vi "rsidr_core_global.vi"() -> ()   [LabVIEW 2020, in "Rohde&Schwarz CMWXP NR FR1 Measurement.lvlib"] (continued)
"Command"="FETC:NRS:MEAS{instance}:MEV:MERR:CURR?", "Access"=enum."Read Only", "Range Table"="", "Read Callback"="", "Write Callback"="", "Range Callback"="", "Check Callback"="", "Rngtable Callback"="", "Coerce Callback"="", "Supported Models"="", "Instrument Options"="", "Check Status Callback"="", "Flags"=0, "Help"="Returns the values of the magnitude error bar graphs for the OFDM symbols in the measured slot. The results of the current bar graph are retrieved.\nThere is one pair of magnitude error values per OFDM symbol, returned in the following order:\n<Reliability>, {<Low>, <High>}symbol 0, {<Low>, <High>}symbol 1, ...\n\nReturn values:\n<Reliability>\n decimal\n\n<Low>\n float\nMagnitude error value for low EVM window position.\nDefault unit:  %\n\n<High>\n float\nMagnitude error value for high EVM window position.\nDefault unit:  %\n\nAvailable Repeated Capabilities:\ninstance: i0, i1, i2, i3, i4, i5, i6, i7, i8, i9, i10, i11, i12, i13, i14, i15, i16, i17, i18, i19, i20, i21, i22, i23, i24, i25, i26, i27, i28, i29, i30, i31, i32\r\n\nRemote-control command(s):\nFETCh:NRSub:MEAS<i>:MEValuation:MERRor:CURRent?"}, {"Level"=4, "Class Only"=FALSE, "Identifier"="RSCMWXPNRFR1M_ATTR_FETCH_MULTI_EVAL_MEAS_MAGNITUDE_ERROR_AVERAGE_RESULTS", "Descriptive Name"="Fetch Multi Eval Meas Magnitude Error Average Results", "Data Type"=enum."RawString", "Command"="FETC:NRS:MEAS{instance}:MEV:MERR:AVER?", "Access"=enum."Read Only", "Range Table"="", "Read Callback"="", "Write Callback"="", "Range Callback"="", "Check Callback"="", "Rngtable Callback"="", "Coerce Callback"="", "Supported Models"="", "Instrument Options"="", "Check Status Callback"="", "Flags"=0, "Help"="Returns the values of the magnitude error bar graphs for the OFDM symbols in the measured slot. The results of the average bar graph are retrieved.\nThere is one pair of magnitude error values per OFDM symbol, returned in the following order:\n<Reliability>, {<Low>, <High>}symbol 0, {<Low>, <High>}symbol 1, ...\n\nReturn values:\n<Reliability>\n decimal\n\n<Low>\n float\nMagnitude error value for low EVM window position.\nDefault unit:  %\n\n<High>\n float\nMagnitude error value for high EVM window position.\nDefault unit:  %\n\nAvailable Repeated Capabilities:\ninstance: i0, i1, i2, i3, i4, i5, i6, i7, i8, i9, i10, i11, i12, i13, i14, i15, i16, i17, i18, i19, i20, i21, i22, i23, i24, i25, i26, i27, i28, i29, i30, i31, i32\r\n\nRemote-control command(s):\nFETCh:NRSub:MEAS<i>:MEValuation:MERRor:AVERage?"}, {"Level"=4, "Class Only"=FALSE, "Identifier"="RSCMWXPNRFR1M_ATTR_FETCH_MULTI_EVAL_MEAS_MAGNITUDE_ERROR_MAXIMUM_RESULTS", "Descriptive Name"="Fetch Multi Eval Meas Magnitude Error Maximum Results", "Data Type"=enum."RawString", "Command"="FETC:NRS:MEAS{instance}:MEV:MERR:MAX?", "Access"=enum."Read Only", "Range Table"="", "Read Callback"="", "Write Callback"="", "Range Callback"="", "Check Callback"="", "Rngtable Callback"="", "Coerce Callback"="", "Supported Models"="", "Instrument Options"="", "Check Status Callback"="", "Flags"=0, "Help"="Returns the values of the magnitude error bar graphs for the OFDM symbols in the measured slot. The results of the maximum bar graph are retrieved.\nThere is one pair of magnitude error values per OFDM symbol, returned in the following order:\n<Reliability>, {<Low>, <High>}symbol 0, {<Low>, <High>}symbol 1, ...\n\nReturn values:\n<Reliability>\n decimal\n\n<Low>\n float\nMagnitude error value for low EVM window position.\nDefault unit:  %\n\n<High>\n float\nMagnitude error value for high EVM window position.\nDefault unit:  %\n\nAvailable Repeated Capabilities:\ninstance: i0, i1, i2, i3, i4, i5, i6, i7, i8, i9, i10, i11, i12, i13, i14, i15, i16, i17, i18, i19, i20, i21, i22, i23, i24, i25, i26, i27, i28, i29, i30, i31, i32\r\n\nRemote-control command(s):\nFETCh:NRSub:MEAS<i>:MEValuation:MERRor:MAXimum?"}, {"Level"=3, "Class Only"=TRUE, "Identifier"="", "Descriptive Name"="Phase Error", "Data Type"=enum."ViInt32", "Command"="", "Access"=enum."Read Only", "Range Table"="", "Read Callback"="", "Write Callback"="", "Range Callback"="", "Check Callback"="", "Rngtable Callback"="", "Coerce Callback"="", "Supported Models"="", "Instrument Options"="", "Check Status Callback"="", "Flags"=0, "Help"="The commands in this class return the contents of the phase error vs OFDM symbol result diagram."}, {"Level"=4, "Class Only"=FALSE, "Identifier"="RSCMWXPNRFR1M_ATTR_READ_MULTI_EVAL_MEAS_PHASE_ERROR_CURRENT_RESULTS", "Descriptive Name"="Read Multi Eval Meas Phase Error Current Results", "Data Type"=enum."RawString", "Command"="READ:NRS:MEAS{instance}:MEV:PERR:CURR?", "Access"=enum."Read Only", "Range Table"="", "Read Callback"="", "Write Callback"="", "Range Callback"="", "Check Callback"="", "Rngtable Callback"="", "Coerce Callback"="", "Supported Models"="", "Instrument Options"="", "Check Status Callback"="", "Flags"=0, "Help"="Returns the values of the phase error bar graphs for the OFDM symbols in the measured slot. The results of the current bar graph are retrieved.\nThere is one pair of phase error values per OFDM symbol, returned in the following order:\n<Reliability>, {<Low>, <High>}symbol 0, {<Low>, <High>}symbol 1, ...\n\nReturn values:\n<Reliability>\n decimal\n\n<Low>\n float\nPhase error value for low EVM window position.\nDefault unit:  deg\n\n<High>\n float\nPhase error value for high EVM window position.\nDefault unit:  deg\n\nAvailable Repeated Capabilities:\ninstance: i0, i1, i2, i3, i4, i5, i6, i7, i8, i9, i10, i11, i12, i13, i14, i15, i16, i17, i18, i19, i20, i21, i22, i23, i24, i25, i26, i27, i28, i29, i30, i31, i32\r\n\nRemote-control command(s):\nREAD:NRSub:MEAS<i>:MEValuation:PERRor:CURRent?"}, {"Level"=4, "Class Only"=FALSE, "Identifier"="RSCMWXPNRFR1M_ATTR_READ_MULTI_EVAL_MEAS_PHASE_ERROR_AVERAGE_RESULTS", "Descriptive Name"="Read Multi Eval Meas Phase Error Average Results", "Data Type"=enum."RawString", "Command"="READ:NRS:MEAS{instance}:MEV:PERR:AVER?", "Access"=enum."Read Only", "Range Table"="", "Read Callback"="", "Write Callback"="", "Range Callback"="", "Check Callback"="", "Rngtable Callback"="", "Coerce Callback"="", "Supported Models"="", "Instrument Options"="", "Check Status Callback"="", "Flags"=0, "Help"="Returns the values of the phase error bar graphs for the OFDM symbols in the measured slot. The results of the average bar graph are retrieved.\nThere is one pair of phase error values per OFDM symbol, returned in the following order:\n<Reliability>, {<Low>, <High>}symbol 0, {<Low>, <High>}symbol 1, ...\n\nReturn values:\n<Reliability>\n decimal\n\n<Low>\n float\nPhase error value for low EVM window position.\nDefault unit:  deg\n\n<High>\n float\nPhase error value for high EVM window position.\nDefault unit:  deg\n\nAvailable Repeated Capabilities:\ninstance: i0, i1, i2, i3, i4, i5, i6, i7, i8, i9, i10, i11, i12, i13, i14, i15, i16, i17, i18, i19, i20, i21, i22, i23, i24, i25, i26, i27, i28, i29, i30, i31, i32\r\n\nRemote-control command(s):\nREAD:NRSub:MEAS<i>:MEValuation:PERRor:AVERage?"}, {"Level"=4, "Class Only"=FALSE, "Identifier"="RSCMWXPNRFR1M_ATTR_READ_MULTI_EVAL_MEAS_PHASE_ERROR_MAXIMUM_RESULTS", "Descriptive Name"="Read Multi Eval Meas Phase Error Maximum Results", "Data Type"=enum."RawString", "Command"="READ:NRS:MEAS{instance}:MEV:PERR:MAX?", "Access"=enum."Read Only", "Range Table"="", "Read Callback"="", "Write Callback"="", "Range Callback"="", "Check Callback"="", "Rngtable Callback"="", "Coerce Callback"="", "Supported Models"="", "Instrument Options"="", "Check Status Callback"="", "Flags"=0, "Help"="Returns the values of the phase error bar graphs for the OFDM symbols in the measured slot. The results of the maximum bar graph are retrieved.\nThere is one pair of phase error values per OFDM symbol, returned in the following order:\n<Reliability>, {<Low>, <High>}symbol 0, {<Low>, <High>}symbol 1, ...\n\nReturn values:\n<Reliability>\n decimal\n\n<Low>\n float\nPhase error value for low EVM window position.\nDefault unit:  deg\n\n<High>\n float\nPhase error value for high EVM window position.\nDefault unit:  deg\n\nAvailable Repeated Capabilities:\ninstance: i0, i1, i2, i3, i4, i5, i6, i7, i8, i9, i10, i11, i12, i13, i14, i15, i16, i17, i18, i19, i20, i21, i22, i23, i24, i25, i26, i27, i28, i29, i30, i31, i32\r\n\nRemote-control command(s):\nREAD:NRSub:MEAS<i>:MEValuation:PERRor:MAXimum?"}, {"Level"=4, "Class Only"=FALSE, "Identifier"="RSCMWXPNRFR1M_ATTR_FETCH_MULTI_EVAL_MEAS_PHASE_ERROR_CURRENT_RESULTS", "Descriptive Name"="Fetch Multi Eval Meas Phase Error Current Results", "Data Type"=enum."RawString", "Command"="FETC:NRS:MEAS{instance}:MEV:PERR:CURR?", "Access"=enum."Read Only", "Range Table"="", "Read Callback"="", "Write Callback"="", "Range Callback"="", "Check Callback"="", "Rngtable Callback"="", "Coerce Callback"="", "Supported Models"="", "Instrument Options"="", "Check Status Callback"="", "Flags"=0, "Help"="Returns the values of the phase error bar graphs for the OFDM symbols in the measured slot. The results of the current bar graph are retrieved.\nThere is one pair of phase error values per OFDM symbol, returned in the following order:\n<Reliability>, {<Low>, <High>}symbol 0, {<Low>, <High>}symbol 1, ...\n\nReturn values:\n<Reliability>\n decimal\n\n<Low>\n float\nPhase error value for low EVM window position.\nDefault unit:  deg\n\n<High>\n float\nPhase error value for high EVM window position.\nDefault unit:  deg\n\nAvailable Repeated Capabilities:\ninstance: i0, i1, i2, i3, i4, i5, i6, i7, i8, i9, i10, i11, i12, i13, i14, i15, i16, i17, i18, i19, i20, i21, i22, i23, i24, i25, i26, i27, i28, i29, i30, i31, i32\r\n\nRemote-control command(s):\nFETCh:NRSub:MEAS<i>:MEValuation:PERRor:CURRent?"}, {"Level"=4, "Class Only"=FALSE, "Identifier"="RSCMWXPNRFR1M_ATTR_FETCH_MULTI_EVAL_MEAS_PHASE_ERROR_AVERAGE_RESULTS", "Descriptive Name"="Fetch Multi Eval Meas Phase Error Average Results", "Data Type"=enum."RawString", "Command"="FETC:NRS:MEAS{instance}:MEV:PERR:AVER?", "Access"=enum."Read Only", "Range Table"="", "Read Callback"="", "Write Callback"="", "Range Callback"="", "Check Callback"="", "Rngtable Callback"="", "Coerce Callback"="", "Supported Models"="", "Instrument Options"="", "Check Status Callback"="", "Flags"=0, "Help"="Returns the values of the phase error bar graphs for the OFDM symbols in the measured slot. The results of the average bar graph are retrieved.\nThere is one pair of phase error values per OFDM symbol, returned in the following order:\n<Reliability>, {<Low>, <High>}symbol 0, {<Low>, <High>}symbol 1, ...\n\nReturn values:\n<Reliability>\n decimal\n\n<Low>\n float\nPhase error value for low EVM window position.\nDefault unit:  deg\n\n<High>\n float\nPhase error value for high EVM window position.\nDefault unit:  deg\n\nAvailable Repeated Capabilities:\ninstance: i0, i1, i2, i3, i4, i5, i6, i7, i8, i9, i10, i11, i12, i13, i14, i15, i16, i17, i18, i19, i20, i21, i22, i23, i24, i25, i26, i27, i28, i29, i30, i31, i32\r\n\nRemote-control command(s):\nFETCh:NRSub:MEAS<i>:MEValuation:PERRor:AVERage?"}, {"Level"=4, "Class Only"=FALSE, "Identifier"="RSCMWXPNRFR1M_ATTR_FETCH_MULTI_EVAL_MEAS_PHASE_ERROR_MAXIMUM_RESULTS", "Descriptive Name"="Fetch Multi Eval Meas Phase Error Maximum Results", "Data Type"=enum."RawString", "Command"="FETC:NRS:MEAS{instance}:MEV:PERR:MAX?", "Access"=enum."Read Only", "Range Table"="", "Read Callback"="", "Write Callback"="", "Range Callback"="", "Check Callback"="", "Rngtable Callback"="", "Coerce Callback"="", "Supported Models"="", "Instrument Options"="", "Check Status Callback"="", "Flags"=0, "Help"="Returns the values of the phase error bar graphs for the OFDM symbols in the measured slot. The results of the maximum bar graph are retrieved.\nThere is one pair of phase error values per OFDM symbol, returned in the following order:\n<Reliability>, {<Low>, <High>}symbol 0, {<Low>, <High>}symbol 1, ...\n\nReturn values:\n<Reliability>\n decimal\n\n<Low>\n float\nPhase error value for low EVM window position.\nDefault unit:  deg\n\n<High>\n float\nPhase error value for high EVM window position.\nDefault unit:  deg\n\nAvailable Repeated Capabilities:\ninstance: i0, i1, i2, i3, i4, i5, i6, i7, i8, i9, i10, i11, i12, i13, i14, i15, i16, i17, i18, i19, i20, i21, i22, i23, i24, i25, i26, i27, i28, i29, i30, i31, i32\r\n\nRemote-control command(s):\nFETCh:NRSub:MEAS<i>:MEValuation:PERRor:MAXimum?"}, {"Level"=3, "Class Only"=TRUE, "Identifier"="", "Descriptive Name"="Inband Emission", "Data Type"=enum."ViInt32", "Command"="", "Access"=enum."Read Only", "Range Table"="", "Read Callback"="", "Write Callback"="", "Range Callback"="", "Check Callback"="", "Rngtable Callback"="", "Coerce Callback"="", "Supported Models"="", "Instrument Options"="", "Check Status Callback"="", "Flags"=0, "Help"="The commands in this class return the inband emission results."}, {"Level"=4, "Class Only"=FALSE, "Identifier"="RSCMWXPNRFR1M_ATTR_READ_MULTI_EVAL_MEAS_TRACE_IEM_CURRENT_RESULTS", "Descriptive Name"="Read Multi Eval Meas Trace IEM Current Results", "Data Type"=enum."RawString", "Command"="READ:NRS:MEAS{instance}:MEV:TRAC:IEM?", "Access"=enum."Read Only", "Range Table"="", "Read Callback"="", "Write Callback"="", "Range Callback"="", "Check Callback"="", "Rngtable Callback"="", "Coerce Callback"="", "Supported Models"="", "Instrument Options"="", "Check Status Callback"="", "Flags"=0, "Help"="Returns the values of the inband emissions trace. The current trace is retrieved.\n\nReturn values:\n<Reliability>\n decimal\n\n<Power>\n float\nComma-separated list of power values, one value per resource block\nDefault unit:  dB\n\nAvailable Repeated Capabilities:\ninstance: i0, i1, i2, i3, i4, i5, i6, i7, i8, i9, i10, i11, i12, i13, i14, i15, i16, i17, i18, i19, i20, i21, i22, i23, i24, i25, i26, i27, i28, i29, i30, i31, i32\r\n\nRemote-control command(s):\nREAD:NRSub:MEAS<i>:MEValuation:TRACe:IEMissions[:CURRent]?"}, {"Level"=4, "Class Only"=FALSE, "Identifier"="RSCMWXPNRFR1M_ATTR_READ_MULTI_EVAL_MEAS_TRACE_IEM_AVERAGE_RESULTS", "Descriptive Name"="Read Multi Eval Meas Trace IEM Average Results", "Data Type"=enum."RawString", "Command"="READ:NRS:MEAS{instance}:MEV:TRAC:IEM:AVER?", "Access"=enum."Read Only", "Range Table"="", "Read Callback"="", "Write Callback"="", "Range Callback"="", "Check Callback"="", "Rngtable Callback"="", "Coerce Callback"="", "Supported Models"="", "Instrument Options"="", "Check Status Callback"="", "Flags"=0, "Help"="Returns the values of the inband emissions trace. The average trace is retrieved.\n\nReturn values:\n<Reliability>\n decimal\n\n<Power>\n float\nComma-separated list of power values, one value per resource block\nDefault unit:  dB\n\nAvailable Repeated Capabilities:\ninstance: i0, i1, i2, i3, i4, i5, i6, i7, i8, i9, i10, i11, i12, i13, i14, i15, i16, i17, i18, i19, i20, i21, i22, i23, i24, i25, i26, i27, i28, i29, i30, i31, i32\r\n\nRemote-control command(s):\nREAD:NRSub:MEAS<i>:MEValuation:TRACe:IEMissions:AVERage?"}, {"Level"=4, "Class Only"=FALSE, "Identifier"="RSCMWXPNRFR1M_ATTR_READ_MULTI_EVAL_MEAS_TRACE_IEM_MAXIMUM_RESULTS", "Descriptive Name"="Read Multi Eval Meas Trace IEM Maximum Results", "Data Type"=enum."RawString", "Command"="READ:NRS:MEAS{instance}:MEV:TRAC:IEM:MAX?", "Access"=enum."Read Only", "Range Table"="", "Read Callback"="", "Write Callback"="", "Range Callback"="", "Check Callback"="", "Rngtable Callback"="", "Coerce Callback"="", "Supported Models"="", "Instrument Options"="", "Check Status Callback"="", "Flags"=0, "Help"="Returns the values of the inband emissions trace. The maximum trace is retrieved.\n\nReturn values:\n<Reliability>\n decimal\n\n<Power>\n float\nComma-separated list of power values, one value per resource block\nDefault unit:  dB\n\nAvailable Repeated Capabilities:\ninstance: i0, i1, i2, i3, i4, i5, i6, i7, i8, i9, i10, i11, i12, i13, i14, i15, i16, i17, i18, i19, i20, i21, i22, i23, i24, i25, i26, i27, i28, i29, i30, i31, i32\r\n\nRemote-control command(s):\nREAD:NRSub:MEAS<i>:MEValuation:TRACe:IEMissions:MAXimum?"}, {"Level"=4, "Class Only"=FALSE, "Identifier"="RSCMWXPNRFR1M_ATTR_FETCH_MULTI_EVAL_MEAS_TRACE_IEM_CURRENT_RESULTS", "Descriptive Name"="Fetch Multi Eval Meas Trace IEM Current Results", "Data Type"=enum."RawString", "Command"="FETC:NRS:MEAS{instance}:MEV:TRAC:IEM?", "Access"=enum."Read Only", "Range Table"="", "Read Callback"="", "Write Callback"="", "Range Callback"="", "Check Callback"="", "Rngtable Callback"="", "Coerce Callback"="", "Supported Models"="", "Instrument Options"="", "Check Status Callback"="", "Flags"=0, "Help"="Returns the values of the inband emissions trace. The current trace is retrieved.\n\nReturn values:\n<Reliability>\n decimal\n\n<Power>\n float\nComma-separated list of power values, one value per resource block\nDefault unit:  dB\n\nAvailable Repeated Capabilities:\ninstance: i0, i1, i2, i3, i4, i5, i6, i7, i8, i9, i10, i11, i12, i13, i14, i15, i16, i17, i18, i19, i20, i21, i22, i23, i24, i25, i26, i27, i28, i29, i30, i31, i32\r\n\nRemote-control command(s):\nFETCh:NRSub:MEAS<i>:MEValuation:TRACe:IEMissions[:CURRent]?"}, {"Level"=4, "Class Only"=FALSE, "Identifier"="RSCMWXPNRFR1M_ATTR_FETCH_MULTI_EVAL_MEAS_TRACE_IEM_AVERAGE_RESULTS", "Descriptive Name"="Fetch Multi Eval Meas Trace IEM Average Results", "Data Type"=enum."RawString", "Command"="FETC:NRS:MEAS{instance}:MEV:TRAC:IEM:AVER?", "Access"=enum."Read Only", "Range Table"="", "Read Callback"="", "Write Callback"="", "Range Callback"="", "Check Callback"="", "Rngtable Callback"="", "Coerce Callback"="", "Supported Models"="", "Instrument Options"="", "Check Status Callback"="", "Flags"=0, "Help"="Returns the values of the inband emissions trace. The average trace is retrieved.\n\nReturn values:\n<Reliability>\n decimal\n\n<Power>\n float\nComma-separated list of power values, one value per resource block\nDefault unit:  dB\n\nAvailable Repeated Capabilities:\ninstance: i0, i1, i2, i3, i4, i5, i6, i7, i8, i9, i10, i11, i12, i13, i14, i15, i16, i17, i18, i19, i20, i21, i22, i23, i24, i25, i26, i27, i28, i29, i30, i31, i32\r\n\nRemote-control command(s):\nFETCh:NRSub:MEAS<i>:MEValuation:TRACe:IEMissions:AVERage?"}, {"Level"=4, "Class Only"=FALSE, "Identifier"="RSCMWXPNRFR1M_ATTR_FETCH_MULTI_EVAL_MEAS_TRACE_IEM_MAXIMUM_RESULTS", "Descriptive Name"="Fetch Multi Eval Meas Trace IEM Maximum Results", "Data Type"=enum."RawString", "Command"="FETC:NRS:MEAS{instance}:MEV:TRAC:IEM:MAX?", "Access"=enum."Read Only", "Range Table"="", "Read Callback"="", "Write Callback"="", "Range Callback"="", "Check Callback"="", "Rngtable Callback"="", "Coerce Callback"="", "Supported Models"="", "Instrument Options"="", "Check Status Callback"="", "Flags"=0, "Help"="Returns the values of the inband emissions trace. The maximum trace is retrieved.\n\nReturn values:\n<Reliability>\n decimal\n\n<Power>\n float\nComma-separated list of power values, one value per resource block\nDefault unit:  dB\n\nAvailable Repeated Capabilities:\ninstance: i0, i1, i2, i3, i4, i5, i6, i7, i8, i9, i10, i11, i12, i13, i14, i15, i16, i17, i18, i19, i20, i21, i22, i23, i24, i25, i26, i27, i28, i29, i30, i31, i32\r\n\nRemote-control command(s):\nFETCh:NRSub:MEAS<i>:MEValuation:TRACe:IEMissions:MAXimum?"}, {"Level"=4, "Class Only"=FALSE, "Identifier"="RSCMWXPNRFR1M_ATTR_READ_MULTI_EVAL_MEAS_TRACE_IEM_LIMIT", "Descriptive Name"="Read Multi Eval Meas Trace IEM Limit", "Data Type"=enum."RawString", "Command"="READ:NRS:MEAS{instance}:MEV:TRAC:IEM:LIM?", "Access"=enum."Read Only", "Range Table"="", "Read Callback"="", "Write Callback"="", "Range Callback"="", "Check Callback"="", "Rngtable Callback"="", "Coerce Callback"="", "Supported Models"="", "Instrument Options"="", "Check Status Callback"="", "Flags"=0, "Help"="Returns the values of the inband emissions limit line.\n\nReturn values:\n<Reliability>\n decimal\n\n<Limit>\n float\nComma-separated list of limit values, one value per resource block\nDefault unit:  dB\n\nAvailable Repeated Capabilities:\ninstance: i0, i1, i2, i3, i4, i5, i6, i7, i8, i9, i10, i11, i12, i13, i14, i15, i16, i17, i18, i19, i20, i21, i22, i23, i24, i25, i26, i27, i28, i29, i30, i31, i32\r\n\nRemote-control command(s):\nREAD:NRSub:MEAS<i>:MEValuation:TRACe:IEMissions:LIMit?"}, {"Level"=4, "Class Only"=FALSE, "Identifier"="RSCMWXPNRFR1M_ATTR_FETCH_MULTI_EVAL_MEAS_TRACE_IEM_LIMIT", "Descriptive Name"="Fetch Multi Eval Meas Trace IEM Limit", "Data Type"=enum."RawString", "Command"="FETC:NRS:MEAS{instance}:MEV:TRAC:IEM:LIM?", "Access"=enum."Read Only", "Range Table"="", "Read Callback"="", "Write Callback"="", "Range Callback"="", "Check Callback"="", "Rngtable Callback"="", "Coerce Callback"="", "Supported Models"="", "Instrument Options"="", "Check Status Callback"="", "Flags"=0, "Help"="Returns the values of the inband emissions limit line.\n\nReturn values:\n<Reliability>\n decimal\n\n<Limit>\n float\nComma-separated list of limit values, one value per resource block\nDefault unit:  dB\n\nAvailable Repeated Capabilities:\ninstance: i0, i1, i2, i3, i4, i5, i6, i7, i8, i9, i10, i11, i12, i13, i14, i15, i16, i17, i18, i19, i20, i21, i22, i23, i24, i25, i26, i27, i28, i29, i30, i31, i32\r\n\nRemote-control command(s):\nFETCh:NRSub:MEAS<i>:MEValuation:TRACe:IEMissions:LIMit?"}, {"Level"=4, "Class Only"=FALSE, "Identifier"="RSCMWXPNRFR1M_ATTR_FETCH_MULTI_EVAL_MEAS_IEM_MARGIN_CURRENT_RESULTS", "Descriptive Name"="Fetch Multi Eval Meas IEM Margin Current Results", "Data Type"=enum."RawString", "Command"="FETC:NRS:MEAS{instance}:MEV:IEM:MARG:CURR?", "Access"=enum."Read Only", "Range Table"="", "Read Callback"="", "Write Callback"="", "Range Callback"="", "Check Callback"="", "Rngtable Callback"="", "Coerce Callback"="", "Supported Models"="", "Instrument Options"="", "Check Status Callback"="", "Flags"=0, "Help"="Return the current limit line margin results. The current margin indicates the minimum (vertical) distance between the inband emissions limit line and the current trace. A negative result indicates that the limit is exceeded. The average, extreme and standard deviation values are calculated from the current margins. The margin results cannot be displayed at the GUI.\n\nReturn values:\n<Reliability>\n decimal\n\n<OutOfTolerance>\n decimal\nOut of tolerance result, i.e. percentage of measurement intervals of the statistic count for modulation measurements exceeding the specified modulation limits.\nDefault unit:  %\n\n<Margin>\n float\nMargin over all non-allocated RBs (scope of general limit component)\nDefault unit:  dB\n\n<IQImage>\n float\nMargin at image frequencies of allocated RBs (scope of IQ image limit component)\nDefault unit:  dB\n\n<CarrLeakage>\n float\nMargin at the carrier frequency (scope of IQ offset limit component)\nDefault unit:  dB\n\nAvailable Repeated Capabilities:\ninstance: i0, i1, i2, i3, i4, i5, i6, i7, i8, i9, i10, i11, i12, i13, i14, i15, i16, i17, i18, i19, i20, i21, i22, i23, i24, i25, i26, i27, i28, i29, i30, i31, i32\r\n\nRemote-control command(s):\nFETCh:NRSub:MEAS<i>:MEValuation:IEMission:MARGin:CURRent?"}, {"Level"=4, "Class Only"=FALSE, "Identifier"="RSCMWXPNRFR1M_ATTR_FETCH_MULTI_EVAL_MEAS_IEM_MARGIN_AVERAGE_RESULTS", "Descriptive Name"="Fetch Multi Eval Meas IEM Margin Average Results", "Data Type"=enum."RawString", "Command"="FETC:NRS:MEAS{instance}:MEV:IEM:MARG:AVER?", "Access"=enum."Read Only", "Range Table"="", "Read Callback"="", "Write Callback"="", "Range Callback"="", "Check Callback"="", "Rngtable Callback"="", "Coerce Callback"="", "Supported Models"="", "Instrument Options"="", "Check Status Callback"="", "Flags"=0, "Help"="Return the average limit line margin results. The current margin indicates the minimum (vertical) distance between the inband emissions limit line and the current trace. A negative result indicates that the limit is exceeded. The average, extreme and standard deviation values are calculated from the current margins. The margin results cannot be displayed at the GUI.\n\nReturn values:\n<Reliability>\n decimal\n\n<OutOfTolerance>\n decimal\nOut of tolerance result, i.e. percentage of measurement intervals of the statistic count for modulation measurements exceeding the specified modulation limits.\nDefault unit:  %\n\n<Margin>\n float\nMargin over all non-allocated RBs (scope of general limit component)\nDefault unit:  dB\n\n<IQImage>\n float\nMargin at image frequencies of allocated RBs (scope of IQ image limit component)\nDefault unit:  dB\n\n<CarrLeakage>\n float\nMargin at the carrier frequency (scope of IQ offset limit component)\nDefault unit:  dB\n\nAvailable Repeated Capabilities:\ninstance: i0, i1, i2, i3, i4, i5, i6, i7, i8, i9, i10, i11, i12, i13, i14, i15, i16, i17, i18, i19, i20, i21, i22, i23, i24, i25, i26, i27, i28, i29, i30, i31, i32\r\n\nRemote-control command(s):\nFETCh:NRSub:MEAS<i>:MEValuation:IEMission:MARGin:AVERage?"}, {"Level"=4, "Class Only"=FALSE, "Identifier"="RSCMWXPNRFR1M_ATTR_FETCH_MULTI_EVAL_MEAS_IEM_MARGIN_EXTREME_RESULTS", "Descriptive Name"="Fetch Multi Eval Meas IEM Margin Extreme Results", "Data Type"=enum."RawString", "Command"="FETC:NRS:MEAS{instance}:MEV:IEM:MARG:EXTR?", "Access"=enum."Read Only", "Range Table"="", "Read Callback"="", "Write Callback"="", "Range Callback"="", "Check Callback"="", "Rngtable Callback"="", "Coerce Callback"="", "Supported Models"="", "Instrument Options"="", "Check Status Callback"="", "Flags"=0, "Help"="Return the extreme limit line margin results. The current margin indicates the minimum (vertical) distance between the inband emissions limit line and the current trace. A negative result indicates that the limit is exceeded. The average, extreme and standard deviation values are calculated from the current margins. The margin results cannot be displayed at the GUI.\n\nReturn values:\n<Reliability>\n decimal\n\n<OutOfTolerance>\n decimal\nOut of tolerance result, i.e. percentage of measurement intervals of the statistic count for modulation measurements exceeding the specified modulation limits.\nDefault unit:  %\n\n<Margin>\n float\nMargin over all non-allocated RBs (scope of general limit component)\nDefault unit:  dB\n\n<IQImage>\n float\nMargin at image frequencies of allocated RBs (scope of IQ image limit component)\nDefault unit:  dB\n\n<CarrLeakage>\n float\nMargin at the carrier frequency (scope of IQ offset limit component)\nDefault unit:  dB\n\nAvailable Repeated Capabilities:\ninstance: i0, i1, i2, i3, i4, i5, i6, i7, i8, i9, i10, i11, i12, i13, i14, i15, i16, i17, i18, i19, i20, i21, i22, i23, i24, i25, i26, i27, i28, i29, i30, i31, i32\r\n\nRemote-control command(s):\nFETCh:NRSub:MEAS<i>:MEValuation:IEMission:MARGin:EXTReme?"}, {"Level"=4, "Class Only"=FALSE, "Identifier"="RSCMWXPNRFR1M_ATTR_FETCH_MULTI_EVAL_MEAS_IEM_MARGIN_STANDARD_DEVIATION_RESULTS", "Descriptive Name"="Fetch Multi Eval Meas IEM Margin Standard Deviation Results", "Data Type"=enum."RawString", "Command"="FETC:NRS:MEAS{instance}:MEV:IEM:MARG:SDEV?", "Access"=enum."Read Only", "Range Table"="", "Read Callback"="", "Write Callback"="", "Range Callback"="", "Check Callback"="", "Rngtable Callback"="", "Coerce Callback"="", "Supported Models"="", "Instrument Options"="", "Check Status Callback"="", "Flags"=0, "Help"="Return the standard deviation limit line margin results. The current margin indicates the minimum (vertical) distance between the inband emissions limit line and the current trace. A negative result indicates that the limit is exceeded.\nThe average, extreme and standard deviation values are calculated from the current margins. The margin results cannot be displayed at the GUI.\n\nReturn values:\n<Reliability>\n decimal\n\n<OutOfTolerance>\n decimal\nOut of tolerance result, i.e. percentage of measurement intervals of the statistic count for modulation measurements exceeding the specified modulation limits.\nDefault unit:  %\n\n<Margin>\n float\nMargin over all non-allocated RBs (scope of general limit component)\nDefault unit:  dB\n\n<IQImage>\n float\nMargin at image frequencies of allocated RBs (scope of IQ image limit component)\nDefault unit:  dB\n\n<CarrLeakage>\n float\nMargin at the carrier frequency (scope of IQ offset limit component)\nDefault unit:  dB\n\nAvailable Repeated Capabilities:\ninstance: i0, i1, i2, i3, i4, i5, i6, i7, i8, i9, i10, i11, i12, i13, i14, i15, i16, i17, i18, i19, i20, i21, i22, i23, i24, i25, i26, i27, i28, i29, i30, i31, i32\r\n\nRemote-control command(s):\nFETCh:NRSub:MEAS<i>:MEValuation:IEMission:MARGin:SDEViation?"}, {"Level"=4, "Class Only"=FALSE, "Identifier"="RSCMWXPNRFR1M_ATTR_FETCH_MULTI_EVAL_MEAS_IEM_MARGIN_RB_INDEX_CURRENT_RESULTS", "Descriptive Name"="Fetch Multi Eval Meas IEM Margin RB Index Current Results", "Data Type"=enum."RawString", "Command"="FETC:NRS:MEAS{instance}:MEV:IEM:MARG:CURR:RBIN?", "Access"=enum."Read Only", "Range Table"="", "Read Callback"="", "Write Callback"="", "Range Callback"="", "Check Callback"="", "Rngtable Callback"="", "Coerce Callback"="", "Supported Models"="", "Instrument Options"="", "Check Status Callback"="", "Flags"=0, "Help"="Return resource block indices for current inband emission margins. At these RB indices, the current, average and extreme margins have been detected.\n\nReturn values:\n<Reliability>\n decimal\n\n<OutOfTolerance>\n decimal\nOut of tolerance result, i.e. percentage of measurement intervals of the statistic count for modulation measurements exceeding the specified modulation limits.\nDefault unit:  %\n\n<RBindex>\n decimal\nResource block index for the general margin (at non-allocated RBs)\n\n<IQImage>\n decimal\nResource block index for the IQ image margin (at image frequencies of allocated RBs)\n\n<CarrLeakage>\n decimal\nResource block index for the carrier leakage margin (at carrier frequency)\n\nAvailable Repeated Capabilities:\ninstance: i0, i1, i2, i3, i4, i5, i6, i7, i8, i9, i10, i11, i12, i13, i14, i15, i16, i17, i18, i19, i20, i21, i22, i23, i24, i25, i26, i27, i28, i29, i30, i31, i32\r\n\nRemote-control command(s):\nFETCh:NRSub:MEAS<i>:MEValuation:IEMission:MARGin:CURRent:RBINdex?"}, {"Level"=4, "Class Only"=FALSE, "Identifier"="RSCMWXPNRFR1M_ATTR_FETCH_MULTI_EVAL_MEAS_IEM_MARGIN_RB_INDEX_AVERAGE_RESULTS", "Descriptive Name"="Fetch Multi Eval Meas IEM Margin RB Index Average Results", "Data Type"=enum."RawString", "Command"="FETC:NRS:MEAS{instance}:MEV:IEM:MARG:AVER:RBIN?", "Access"=enum."Read Only", "Range Table"="", "Read Callback"="", "Write Callback"="", "Range Callback"="", "Check Callback"="", "Rngtable Callback"="", "Coerce Callback"="", "Supported Models"="", "Instrument Options"="", "Check Status Callback"="", "Flags"=0, "Help"="Return resource block indices for average inband emission margins. At these RB indices, the current, average and extreme margins have been detected.\n\nReturn values:\n<Reliability>\n decimal\n\n<OutOfTolerance>\n decimal\nOut of tolerance result, i.e. percentage of measurement intervals of the statistic count for modulation measurements exceeding the specified modulation limits.\nDefault unit:  %\n\n<RBindex>\n decimal\nResource block index for the general margin (at non-allocated RBs)\n\n<IQImage>\n decimal\nResource block index for the IQ image margin (at image frequencies of allocated RBs)\n\n<CarrLeakage>\n decimal\nResource block index for the carrier leakage margin (at carrier frequency)\n\nAvailable Repeated Capabilities:\ninstance: i0, i1, i2, i3, i4, i5, i6, i7, i8, i9, i10, i11, i12, i13, i14, i15, i16, i17, i18, i19, i20, i21, i22, i23, i24, i25, i26, i27, i28, i29, i30, i31, i32\r\n\nRemote-control command(s):\nFETCh:NRSub:MEAS<i>:MEValuation:IEMission:MARGin:AVERage:RBINdex?"}, {"Level"=4, "Class Only"=FALSE, "Identifier"="RSCMWXPNRFR1M_ATTR_FETCH_MULTI_EVAL_MEAS_IEM_MARGIN_RB_INDEX_EXTREME_RESULTS", "Descriptive Name"="Fetch Multi Eval Meas IEM Margin RB Index Extreme Results", "Data Type"=enum."RawString", "Command"="FETC:NRS:MEAS{instance}:MEV:IEM:MARG:EXTR:RBIN?", "Access"=enum."Read Only", "Range Table"="", "Read Callback"="", "Write Callback"="", "Range Callback"="", "Check Callback"="", "Rngtable Callback"="", "Coerce Callback"="", "Supported Models"="", "Instrument Options"="", "Check Status Callback"="", "Flags"=0, "Help"="Return resource block indices for extreme inband emission margins. At these RB indices, the current, average and extreme margins have been detected.\n\nReturn values:\n<Reliability>\n decimal\n\n<OutOfTolerance>\n decimal\nOut of tolerance result, i.e. percentage of measurement intervals of the statistic count for modulation measurements exceeding the specified modulation limits.\nDefault unit:  %\n\n<RBindex>\n decimal\nResource block index for the general margin (at non-allocated RBs)\n\n<IQImage>\n decimal\nResource block index for the IQ image margin (at image frequencies of allocated RBs)\n\n<CarrLeakage>\n decimal\nResource block index for the carrier leakage margin (at carrier frequency)\n\nAvailable Repeated Capabilities:\ninstance: i0, i1, i2, i3, i4, i5, i6, i7, i8, i9, i10, i11, i12, i13, i14, i15, i16, i17, i18, i19, i20, i21, i22, i23, i24, i25, i26, i27, i28, i29, i30, i31, i32\r\n\nRemote-control command(s):\nFETCh:NRSub:MEAS<i>:MEValuation:IEMission:MARGin:EXTReme:RBINdex?"}, {"Level"=3, "Class Only"=TRUE, "Identifier"="", "Descriptive Name"="Equalizer Spectrum Flatness", "Data Type"=enum."ViInt32", "Command"="", "Access"=enum."Read Only", "Range Table"="", "Read Callback"="", "Write Callback"="", "Range Callback"="", "Check Callback"="", "Rngtable Callback"="", "Coerce Callback"="", "Supported Models"="", "Instrument Options"="", "Check Status Callback"="", "Flags"=0, "Help"="The commands in this class return the equalizer spectrum flatness results."}, {"Level"=4, "Class Only"=FALSE, "Identifier"="RSCMWXPNRFR1M_ATTR_READ_MULTI_EVAL_MEAS_TRACE_ES_FLATNESS_RESULTS", "Descriptive Name"="Read Multi Eval Meas Trace ES Flatness Results", "Data Type"=enum."RawString", "Command"="READ:NRS:MEAS{instance}:MEV:TRAC:ESFL?", "Access"=enum."Read Only", "Range Table"="", "Read Callback"="", "Write Callback"="", "Range Callback"="", "Check Callback"="", "Rngtable Callback"="", "Coerce Callback"="", "Supported Models"="", "Instrument Options"="", "Check Status Callback"="", "Flags"=0, "Help"="Returns the values of the equalizer spectrum flatness trace.\n\nReturn values:\n<Reliability>\n decimal\n\n<Power>\n float\nComma-separated list of power values, one value per subcarrier\nFor not allocated subcarriers, NCAP is returned.\nDefault unit:  dB\n\nAvailable Repeated Capabilities:\ninstance: i0, i1, i2, i3, i4, i5, i6, i7, i8, i9, i10, i11, i12, i13, i14, i15, i16, i17, i18, i19, i20, i21, i22, i23, i24, i25, i26, i27, i28, i29, i30, i31, i32\r\n\nRemote-control command(s):\nREAD:NRSub:MEAS<i>:MEValuation:TRACe:ESFLatness?"}, {"Level"=4, "Class Only"=FALSE, "Identifier"="RSCMWXPNRFR1M_ATTR_FETCH_MULTI_EVAL_MEAS_TRACE_ES_FLATNESS_RESULTS", "Descriptive Name"="Fetch Multi Eval Meas Trace ES Flatness Results", "Data Type"=enum."RawString", "Command"="FETC:NRS:MEAS{instance}:MEV:TRAC:ESFL?", "Access"=enum."Read Only", "Range Table"="", "Read Callback"="", "Write Callback"="", "Range Callback"="", "Check Callback"="", "Rngtable Callback"="", "Coerce Callback"="", "Supported Models"="", "Instrument Options"="", "Check Status Callback"="", "Flags"=0, "Help"="Returns the values of the equalizer spectrum flatness trace.\n\nReturn values:\n<Reliability>\n decimal\n\n<Power>\n float\nComma-separated list of power values, one value per subcarrier\nFor not allocated subcarriers, NCAP is returned.\nDefault unit:  dB\n\nAvailable Repeated Capabilities:\ninstance: i0, i1, i2, i3, i4, i5, i6, i7, i8, i9, i10, i11, i12, i13, i14, i15, i16, i17, i18, i19, i20, i21, i22, i23, i24, i25, i26, i27, i28, i29, i30, i31, i32\r\n\nRemote-control command(s):\nFETCh:NRSub:MEAS<i>:MEValuation:TRACe:ESFLatness?"}, {"Level"=4, "Class Only"=FALSE, "Identifier"="RSCMWXPNRFR1M_ATTR_READ_MULTI_EVAL_MEAS_ES_FLATNESS_CURRENT_RESULTS", "Descriptive Name"="Read Multi Eval Meas ES Flatness Current Results", "Data Type"=enum."RawString", "Command"="READ:NRS:MEAS{instance}:MEV:ESFL:CURR?", "Access"=enum."Read Only", "Range Table"="", "Read Callback"="", "Write Callback"="", "Range Callback"="", "Check Callback"="", "Rngtable Callback"="", "Coerce Callback"="", "Supported Models"="", "Instrument Options"="", "Check Status Callback"="", "Flags"=0, "Help"="Return current single value results of the equalizer spectrum flatness measurement.\n\n<1_Reliability>\n decimal\n\n<2_OutOfTol>\n decimal\nOut of tolerance result, i.e. percentage of measurement intervals of the statistic count for modulation measurements exceeding the specified modulation limits.\nDefault unit:  %\n\n<3_Ripple1>\n float\nMax (range 1) - min (range 1)\nDefault unit:  dB\n\n<4_Ripple2>\n float\nMax (range 2) - min (range 2)\nDefault unit:  dB\n\n<5_MaxR1MinR2>\n float\nMax (range 1) - min (range 2)\nDefault unit:  dB\n\n<6_MaxR2MinR1>\n float\nMax (range 2) - min (range 1)\nDefault unit:  dB\n\n<7_MinR1>\n float\nMin (range 1)\nDefault unit:  dB\n\n<8_MaxR1>\n float\nMax (range 1)\nDefault unit:  dB\n\n<9_MinR2>\n float\nMin (range 2)\nDefault unit:  dB\n\n<10_MaxR2>\n float\nMax (range 2)\nDefault unit:  dB\n\nAvailable Repeated Capabilities:\ninstance: i0, i1, i2, i3, i4, i5, i6, i7, i8, i9, i10, i11, i12, i13, i14, i15, i16, i17, i18, i19, i20, i21, i22, i23, i24, i25, i26, i27, i28, i29, i30, i31, i32\r\n\nRemote-control command(s):\nREAD:NRSub:MEAS<i>:MEValuation:ESFLatness:CURRent?"}, {"Level"=4, "Class Only"=FALSE, "Identifier"="RSCMWXPNRFR1M_ATTR_READ_MULTI_EVAL_MEAS_ES_FLATNESS_AVERAGE_RESULTS", "Descriptive Name"="Read Multi Eval Meas ES Flatness Average Results", "Data Type"=enum."RawString", "Command"="READ:NRS:MEAS{instance}:MEV:ESFL:AVER?", "Access"=enum."Read Only", "Range Table"="", "Read Callback"="", "Write Callback"="", "Range Callback"="", "Check Callback"="", "Rngtable Callback"="", "Coerce Callback"="", "Supported Models"="", "Instrument Options"="", "Check Status Callback"="", "Flags"=0, "Help"="Return average single value results of the equalizer spectrum flatness measurement.\n\n<1_Reliability>\n decimal\n\n<2_OutOfTol>\n decimal\nOut of tolerance result, i.e. percentage of measurement intervals of the statistic count for modulation measurements exceeding the specified modulation limits.\nDefault unit:  %\n\n<3_Ripple1>\n float\nMax (range 1) - min (range 1)\nDefault unit:  dB\n\n<4_Ripple2>\n float\nMax (range 2) - min (range 2)\nDefault unit:  dB\n\n<5_MaxR1MinR2>\n float\nMax (range 1) - min (range 2)\nDefault unit:  dB\n\n<6_MaxR2MinR1>\n float\nMax (range 2) - min (range 1)\nDefault unit:  dB\n\n<7_MinR1>\n float\nMin (range 1)\nDefault unit:  dB\n\n<8_MaxR1>\n float\nMax (range 1)\nDefault unit:  dB\n\n<9_MinR2>\n float\nMin (range 2)\nDefault unit:  dB\n\n<10_MaxR2>\n float\nMax (range 2)\nDefault unit:  dB\n\nAvailable Repeated Capabilities:\ninstance: i0, i1, i2, i3, i4, i5, i6, i7, i8, i9, i10, i11, i12, i13, i14, i15, i16, i17, i18, i19, i20, i21, i22, i23, i24, i25, i26, i27, i28, i29, i30, i31, i32\r\n\nRemote-control command(s):\nREAD:NRSub:MEAS<i>:MEValuation:ESFLatness:AVERage?"}, {"Level"=4, "Class Only"=FALSE, "Identifier"="RSCMWXPNRFR1M_ATTR_READ_MULTI_EVAL_MEAS_ES_FLATNESS_EXTREME_RESULTS", "Descriptive Name"="Read Multi Eval Meas ES Flatness Extreme Results", "Data Type"=enum."RawString", "Command"="READ:NRS:MEAS{instance}:MEV:ESFL:EXTR?", "Access"=enum."Read Only", "Range Table"="", "Read Callback"="", "Write Callback"="", "Range Callback"="", "Check Callback"="", "Rngtable Callback"="", "Coerce Callback"="", "Supported Models"="", "Instrument Options"="", "Check Status Callback"="", "Flags"=0, "Help"="Return extreme single value results of the equalizer spectrum flatness measurement.\n\n<1_Reliability>\n decimal\n\n<2_OutOfTol>\n decimal\nOut of tolerance result, i.e. percentage of measurement intervals of the statistic 
